vi "Intake Set.vi"(1 "Intake Info In":T2) -> (0 "Intake Info Out":T2)   [LabVIEW 2013]
uses:
  <vilib>/Rock Robotics/WPI/Solenoid/WPI_SolenoidValue.ctl
  <vilib>/Rock Robotics/WPI/Solenoid/WPI_SolenoidSetEnum.vi
panel:
  # "True = Out\nFalse = In"
  # "True = Out\nFalse = In"
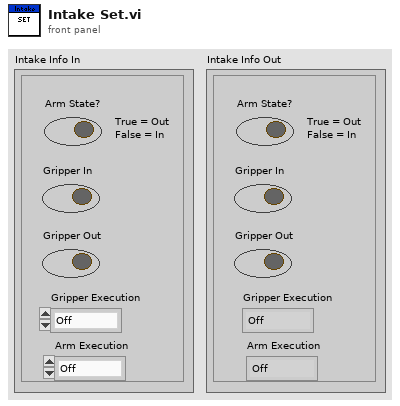
[diagram p1: front panel]
types:
  T1 = typedef "WPI_SolenoidValue.ctl" = enum16{"Off", "On", "Forward", "Reverse"}
  T2 = cluster{"Arm State?":bool, "Gripper In":bool, "Gripper Out":bool, "Gripper Execution ":T1, "Arm Execution ":T1}
  T3 = typedef "WPI_RelayDevRef.ctl" = cluster{"DevStatus":errorcluster, "Relay Channel":T4, "Digital Module":T5, "Relay Direction":T6}
  T4 = typedef "FPGA_DIORelayChannel.ctl" = enum8{"Relay 1", "Relay 2", "Relay 3", "Relay 4", "Relay 5", "Relay 6", "Relay 7", "Relay 8", "Invalid"}
  T5 = typedef "FPGA_TypedefDigitalModule.ctl" = enum16{"Digital Module 1", "Digital Module 2"}
  T6 = typedef "WPI_RelayDirection.ctl" = enum16{"Both directions", "Forward only", "Reverse only"}
  T7 = typedef "WPI_SolenoidDevRef.ctl" = cluster{"DevStatus":errorcluster, "Solenoid Module":T8, "Forward Solenoid Channel":T9, "Reverse Solenoid Channel":T9}
  T8 = typedef "FPGA_TypedefSolenoidModule.ctl" = enum16{"Solenoid Module 1", "Solenoid Module 2"}
  T9 = typedef "WPI_SolenoidChannel.ctl" = enum8{"Solenoid 1", "Solenoid 2", "Solenoid 3", "Solenoid 4", "Solenoid 5", "Solenoid 6", "Solenoid 7", "Solenoid 8", "Invalid"}
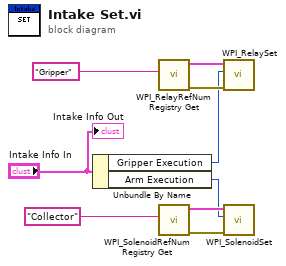
[diagram p0: block diagram]
diagram:
  n1 = Unbundle By Name("Intake Info In") -> ("Gripper Execution"=w1:T1, "Arm Execution"=w2:T1)
  n2 = call <vilib>:"WPI_RelayRefNum Registry Get.vi"("refnum name"="Gripper") -> ("error out"=w6:errorcluster, "RelayDevRef"=w5:T3)  [unwired: 9 in]
  n3 = call <vilib>:"WPI_SolenoidRefNum Registry Get.vi"("refnum name"="Collector") -> ("error out"=w4:errorcluster, "SolenoidDevRef"=w3:T7)  [unwired: 9 in]
  n4 = call <vilib>:"WPI_RelaySet.vi"("error in (no error)"=w6, "RelayValue"=w1, "RelayDevRef"=w5) -> ()  [unwired: 7 in, 2 out]
  n5 = call-poly <vilib>:"WPI_SolenoidSet.vi"("error in (no error)"=w4, "Value"=w2, "SolenoidDevRef"=w3) -> ()  [unwired: 7 in, 2 out]
  "Intake Info Out" <- "Intake Info In"
